vi "Not A Windows Message Queue.vi"(0 "win msg queue":T1, 1 "error in (no error)":errorcluster) -> (2 "win msg queue":T1, 3 "Not a Queue?":bool, 4 "error out":errorcluster)   [LabVIEW 2017, in "Windows messages for Labview (32 and 64).lvlib"]
doc: "Determines whether win msg queue is a valid windows message queue. Returns True if win msg queue is not valid."
uses:
  Windows messages for Labview (32 and 64).lvlib
  Win Msg Queue RefNum.ctl
  Windows Messages for LabVIEW_32.dll
  Windows Messages for LabVIEW_64.dll
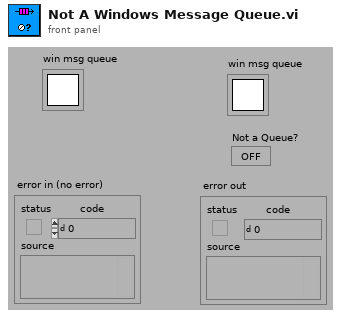
[diagram p1: front panel]
types:
  T1 = typedef "Windows messages for Labview (32 and 64).lvlib/Win Msg Queue RefNum.ctl" = refnum<k1>
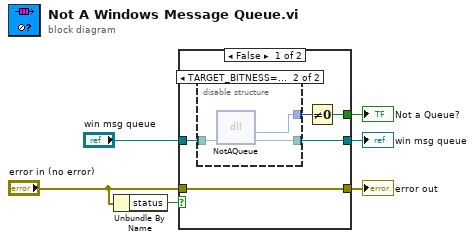
[diagram p0: block diagram]
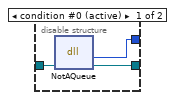
[diagram p2: hidden frame]
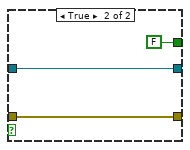
[diagram p3: hidden frame]
diagram:
  n1 = Unbundle By Name("error in (no error)") -> ("status"=w3:bool)
  n2 = case shown="False" w3 {
    tunnel: "win msg queue" -> [w9 w19]
    tunnel: [w10 FALSE] -> w1
    tunnel: "error in (no error)" -> [w11 w20]
    tunnel: [w11 w20] -> w4
    tunnel: [w7 w19] -> w2
    frame False {
      n3 = disable-structure shown="TARGET_BITNESS==32" {
        disable-tunnel: w9 -> [w14 w17]
        disable-tunnel: [w13 w16] -> w7
        disable-tunnel: [w12 w15] -> w8
        frame condition #0 (active) {
          n4 = dll-call lib="M:/_dev/progs/LabVIEW/_lib/Windows Messages for Labview/llb/Windows Messages for LabVIEW_64.dll" fn="NotAQueue"("occurrence"=w14) -> ("return type"=w12:i32, "occurrence"=w13:T1)  [unwired: 3 in, 2 out]
        }
        frame condition #1 {
          n5 = dll-call lib="D:/labview_d/temp/Windows Messaging/Windows Messages for Labview/llb/Windows Messages for LabVIEW_32.dll" fn="NotAQueue"("occurrence"=w17) -> ("return type"=w15:i32, "occurrence"=w16:T1)  [unwired: 3 in, 2 out]
        }
      }
      n6 = Not Equal To 0?(x=w8) -> (x != 0?=w10:bool)
    }
    frame True {
    }
  }
  "error out" <- w4
  "win msg queue" <- w2
  "Not a Queue?" <- w1
